vi "IO.Export.vi"(8 "error in (no error)":errorcluster, 11 "Item Ref in":T1 format="%.0x") -> (0 "error out":errorcluster, 2 "IO":T2 {"Signals"."Response"."Byte Order" items=["Little Endian", "Big Endian"]; "Signals"."Response"."Data Type" items=["Signed", "Unsigned", "IEEE Float"]; "Signals"."Cmd"."Byte Order" items=["Little Endian", "Big Endian"]; "Signals"."Cmd"."Data Type" items=["Signed", "Unsigned", "IEEE Float"]}, 3 "Section Ref out":T1 format="%.0x")   [LabVIEW 2019, in "Diagnostics Addon System Explorer.lvlib"]
uses:
  Diagnostics Addon System Explorer.lvlib
  <vilib>/NI VeriStand/Custom Device API/Custom Device Item Ref.ctl
  Types/IO.Export.ctl
  Types/CmdResp.Export.ctl
  Shared/Types/Signal.ctl
  Types/FG.Action.ctl
  Signals.Get.vi
  Type.FG.vi
  Signal.FG.vi
  Shared/SubVIs/Constants.vi
  <vilib>/NI/NI VeriStand Advanced SysDef API/SysDef API/SysDef.Property.Set.vi
  <vilib>/NI/NI VeriStand Advanced SysDef API/_SubVIs/SysDef.Property.Set.U32.vi
  <vilib>/NI VeriStand/Custom Device API/NI VeriStand - Get Item Property.vi
  <vilib>/NI VeriStand/Custom Device API/Get Item Property (U32).vi
  <vilib>/NI VeriStand/Custom Device Tools/Custom Device Utility Library/NI VeriStand - Search for Item.vi
  <vilib>/NI VeriStand/Custom Device Tools/Custom Device Utility Library/NI VeriStand - Search for Item by GUID.vi
  <vilib>/NI VeriStand/Custom Device API/NI VeriStand - Get Item Children.vi
  <vilib>/NI/NI VeriStand Advanced SysDef API/_SubVIs/SysDef.Property.Set.DBL.vi
  <vilib>/NI/NI VeriStand Advanced SysDef API/_SubVIs/SysDef.Property.Set.String.vi
  <vilib>/NI VeriStand/Custom Device API/Get Item Property (Double).vi
  <vilib>/NI VeriStand/Custom Device API/Get Item Property (String).vi
  <vilib>/NI VeriStand/Custom Device API/NI VeriStand - Get Custom Device Channel Data.vi
  Shared/Diagnostics Addon Shared.lvlib
  <vilib>/NI VeriStand/Custom Device API/Custom Device API.lvlib
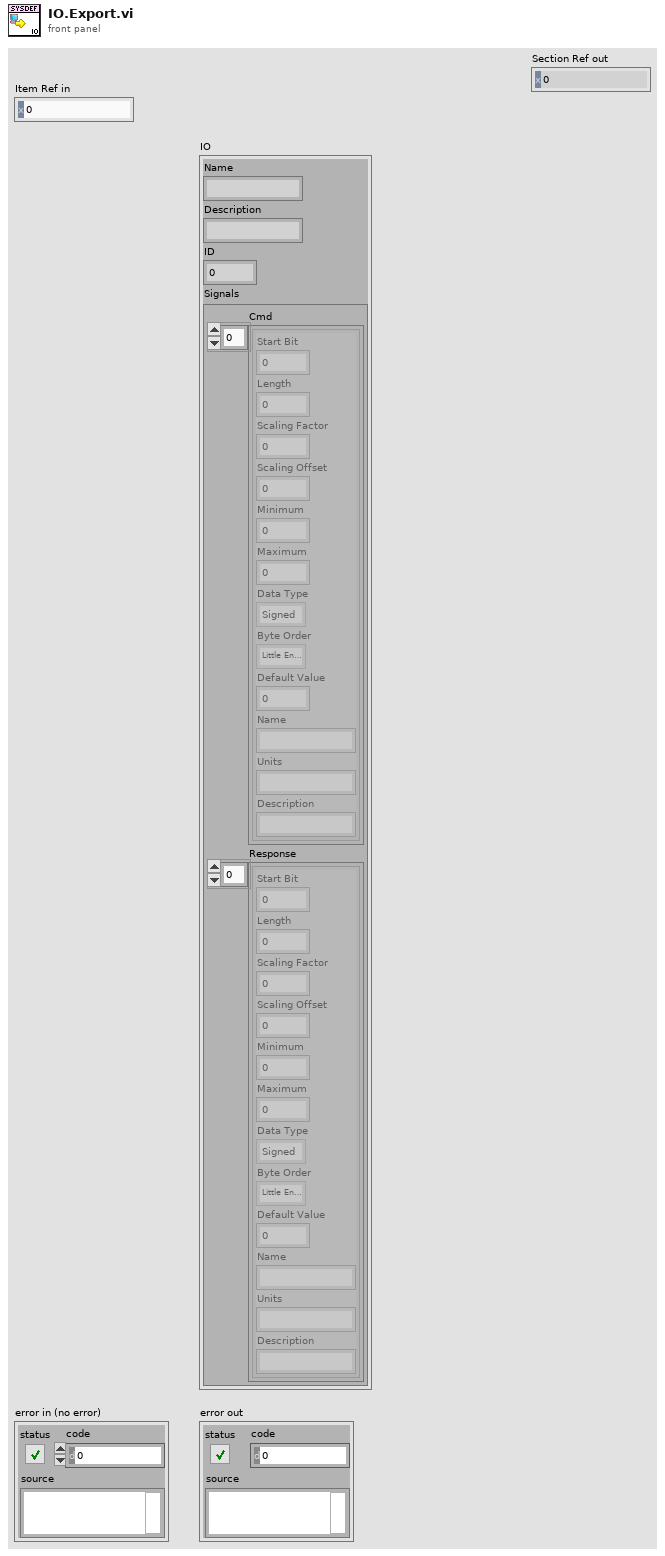
[diagram p1: front panel]
types:
  T1 = typedef "Custom Device API.lvlib/Custom Device Item Ref.ctl" = u64
  T2 = typedef "Diagnostics Addon System Explorer.lvlib/IO.Export.ctl" = cluster{"Name":string, "Description":string, "ID":u16, "Signals":T3}
  T3 = typedef "Diagnostics Addon System Explorer.lvlib/CmdResp.Export.ctl" = cluster{"Cmd":T4[], "Response":T4[]}
  T4 = typedef "Diagnostics Addon Shared.lvlib/Signal.ctl" = cluster{"Start Bit":u32, "Length":u32, "Scaling Factor":dbl, "Scaling Offset":dbl, "Minimum":dbl, "Maximum":dbl, "Data Type":u32, "Byte Order":u32, "Default Value":dbl, "Name":string, "Units":string, "Description":string}
  T5 = typedef "Diagnostics Addon System Explorer.lvlib/FG.Action.ctl" = enum16{"Get", "Set"}
  T6 = typedef "Custom Device API.lvlib/Custom Device Item Info.ctl" = cluster{"Name":string, "Is Channel":bool, "GUID":string, "Is Waveform":bool}
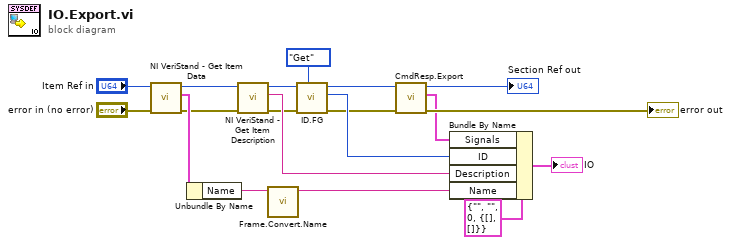
[diagram p0: block diagram]
diagram:
  n1 = call <vilib>:"NI VeriStand - Get Item Data.vi"("error in (no error)"="error in (no error)", "Item Ref in"="Item Ref in") -> ("error out"=w16:errorcluster, "Item Info"=w17:T6, "Item Ref out"=w14:T1)  [unwired: 6 in, 1 out]
  n2 = Unbundle By Name(w17) -> ("Name"=w18:string)
  n3 = call <vilib>:"NI VeriStand - Get Item Description.vi"("error in (no error)"=w16, "Item Ref in"=w14) -> ("error out"=w9:errorcluster, "Description"=w11:string, "Item Ref out"=w10:T1)  [unwired: 6 in, 1 out]
  n4 = call "Frame.Convert.Name.vi"("VS Frame Name"=w18) -> ("Frame Name"=w1:string)  [unwired: 9 in, 1 out]
  n5 = call "ID.FG.vi"("Action"=FG.Action."Get", "error in (no error)"=w9, "Device Item Ref in"=w10) -> ("error out"=w3:errorcluster, "ID"=w12:u32, "Device Item Ref out"=w2:T1)  [unwired: 6 in]
  n6 = call "CmdResp.Export.vi"("error in (no error)"=w3, "Device Item Ref in"=w2) -> ("error out"=→"error out":errorcluster, "Signals"=w5:T3, "Section Ref out"=→"Section Ref out":T1)  [unwired: 7 in]
  n7 = Bundle By Name(cluster=T2 {"Name"="", "Description"="", "ID"=0, "Signals"={"Cmd"=[], "Response"=[]}} ("IO"), "Signals"=w5, "ID"=w12, "Description"=w11, "Name"=w1) -> (→"IO":T2)
